vi "filters.vi"(4 "error in (no error)":errorcluster, 7 "Array":waveform(i16)[](array[waveform])) -> (3 "Array 2":waveform(i16)[](array[waveform]))   [LabVIEW 2010]
uses:
  <vilib>/Analysis/3filter.llb/Filter Passband Type.ctl
  skil/lib/Global 2.vi
  <vilib>/Analysis/3filter.llb/Equi-Ripple HighPass (DBL).vi
  <vilib>/Analysis/3filter.llb/Bessel Filter (DBL).vi
  <vilib>/Waveform/WDTOps.llb/WDT Get Waveform Subset I16.vi
  <vilib>/Utility/config.llb/NI_LVConfig.lvlib
  <vilib>/Analysis/NI_AALBase.lvlib
panel:
  out "Waveform Graph":waveform(i16)[](graph)
  out "error out":errorcluster
  in  "order":i32=3
  in  "high_freq":dbl=500000.0 format="%#_4p"
  in  "stop_freq":dbl=350000.0 format="%#_4p"
  in  "taps":i32=500
  in  "filter":enum16{"none", "Гребёнка", "FIR", "Bessel"}(ring)
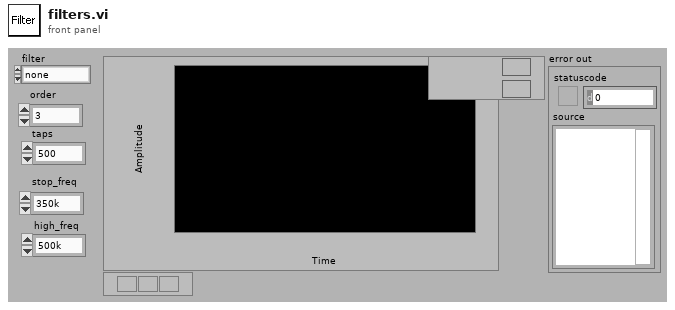
[diagram p1: front panel]
types:
  T1 = typedef "NI_AALBase.lvlib/Filter Passband Type.ctl" = enum32{"Lowpass", "Highpass", "Bandpass", "Bandstop"}
  T2 = typedef "NI_LVConfig.lvlib/Config Data RefNum.ctl" = refnum<k1>
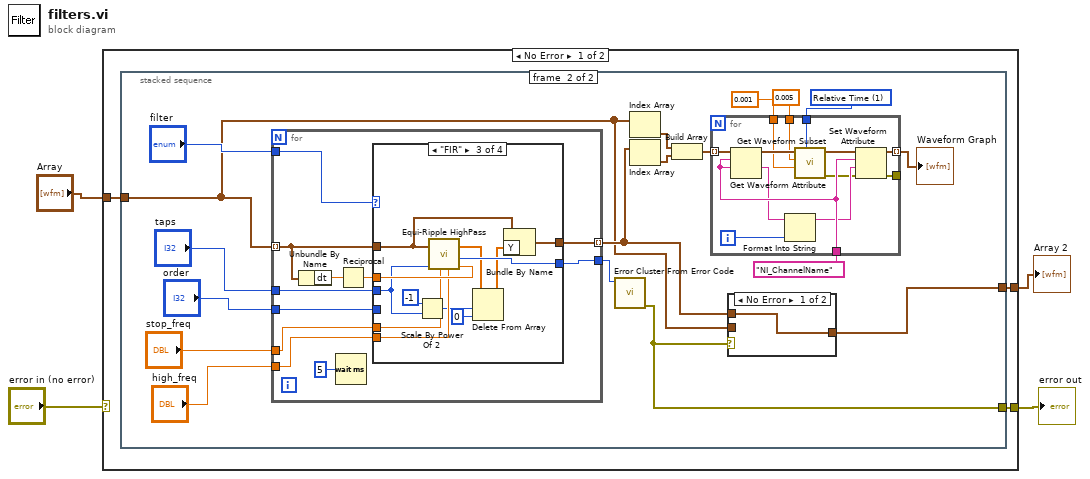
[diagram p0: block diagram]
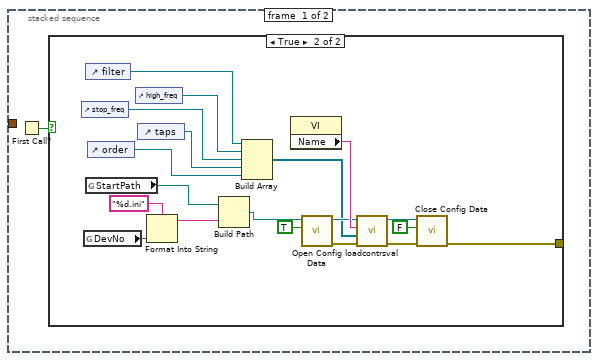
[diagram p2: hidden frame]
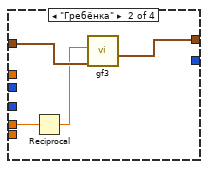
[diagram p6: hidden frame]
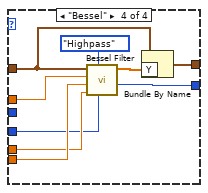
[diagram p7: hidden frame]
diagram:
  n1 = case shown="No Error" "error in (no error)" {
    selector: "error in (no error)" -> [_ w99]
    tunnel: [w7 w99] -> w3
    tunnel: "Array" -> [w6 w98]
    tunnel: [w5 w98] -> w1
    frame No Error {
      n2 = stacked-sequence {
        tunnel: [_ w31] -> w7
        tunnel: w6 -> [_ w29]
        tunnel: [_ w28] -> w5
        frame #0 {
          n3 = First Call?() -> (First Call?: T/F=w8:bool)
          n4 = case shown="True" w8 {
            tunnel: [_ w14] -> _
            frame False {
            }
            frame True {
              n5 = control-ref of="stop_freq"() -> (w11:refnum<vi>)
              n6 = global read "Global 2.vi" "DevNo"() -> (w18:i32)
              n7 = control-ref of="filter"() -> (w13:refnum<vi>)
              n8 = global read "Global 2.vi" "StartPath"() -> (w15:path)
              n9 = control-ref of="order"() -> (w9:refnum<vi>)
              n10 = control-ref of="high_freq"() -> (w12:refnum<vi>)
              n11 = control-ref of="taps"() -> (w10:refnum<vi>)
              n12 = Format Into String(format string="%d.ini", w18) -> (resulting string=w17:string)  [unwired: 2 in, 1 out]
              n13 = Build Path(base path=w15, name or relative path=w17) -> (appended path=w19:path)
              n14 = Build Array(w13, w12, w11, w10, w9) -> (w21:refnum<vi>[])
              n15 = property class="VI"() -> ("Name"=w24:string)  [unwired: 2 in, 2 out]
              n16 = call <vilib>:"Open Config Data.vi"("create file if necessary (T)"=TRUE, "configuration file path"=w19) -> ("error out"=w26:errorcluster, "refnum"=w23:T2)  [unwired: 7 in, 1 out]
              n17 = call "loadcontrsval.vi"("error in"=w26, "Array"=w21, "Section"=w24, "refnum in"=w23) -> ("error out"=w25:errorcluster, "refnum out"=w22:T2)  [unwired: 1 in, 1 out]
              n18 = call <vilib>:"Close Config Data.vi"("error in (no error)"=w25, "write file if changed (T)"=FALSE, "refnum"=w22) -> ("error out"=w14:errorcluster)  [unwired: 7 in, 1 out]
            }
          }
        }
        frame #1 {
          w39 = u16 1 items=["Index", "Relative Time"] ("start/duration format")
          n19 = for {
            tunnel: "filter" -> [w71]
            tunnel: w29 -> [w67] mode=indexing
            tunnel: [w70] -> w30 mode=indexing
            tunnel: [w69] -> w40
            tunnel: "taps" -> [w68]
            tunnel: "stop_freq" -> [w66]
            tunnel: "high_freq" -> [w65]
            tunnel: "order" -> [w64]
            n20 = Unbundle By Name(w67) -> ("dt"=w63:dbl)
            n21 = Wait (ms)(milliseconds to wait=u32 5) -> ()  [unwired: 1 out]
            n22 = Reciprocal(x=w63) -> (1/x=w62:dbl)
            n23 = case shown="\"FIR\"" w71 {
              tunnel: w67 -> [w72 w76 w84 w92]
              tunnel: [w72 w75 w83 w90] -> w70
              tunnel: [_ _ w88 w96] -> w69
              tunnel: w68 -> [_ _ w82 _]
              tunnel: w62 -> [_ _ w87 w95]
              tunnel: w66 -> [_ w74 w86 w93]
              tunnel: w65 -> [_ _ w85 w94]
              tunnel: w64 -> [_ _ _ w89]
              frame "none", Default {
              }
              frame "Гребёнка" {
                n24 = Reciprocal(x=w74) -> (1/x=w73:dbl)
                n25 = call "gf3.vi"("Waveform"=w76, "T"=w73) -> ("Waveform 2"=w75:waveform(i16))  [unwired: 4 in, 1 out]
              }
              frame "FIR" {
                n26 = Scale By Power Of 2(n=-1, x=w82) -> (x*2^n=w80:i32)
                n27 = call-poly <vilib>:"Equi-Ripple HighPass.vi"("# of taps"=w82, "stop freq"=w86, "high freq"=w85, "sampling freq: fs"=w87, "X"=w84) -> ("error"=w88:i32, "Filtered X"=w79:dbl[])  [unwired: 1 in]
                n28 = Delete From Array(array=w79, length=w80, index=0) -> (array with subset deleted=w78:dbl[])  [unwired: 1 out]
                n29 = Bundle By Name(cluster=w84, "Y"=w78) -> (w83:waveform(i16))
              }
              frame "Bessel" {
                n30 = call-poly <vilib>:"Bessel Filter.vi"("order"=w89, "filter type"=Filter_Passband_Type."Highpass", "low cutoff freq: fl"=w93, "high cutoff freq: fh"=w94, "sampling freq: fs"=w95, "X"=w92) -> ("error"=w96:i32, "Filtered X"=w91:dbl[])  [unwired: 2 in]
                n31 = Bundle By Name(cluster=w92, "Y"=w91) -> (w90:waveform(i16))
              }
            }
          }
          n32 = call <vilib>:"Error Cluster From Error Code.vi"("error code (0)"=w40) -> ("error out"=w31:errorcluster)  [unwired: 8 in]
          n33 = Index Array(array=w29) -> (element=w36:waveform(i16))  [unwired: 1 in]
          n34 = Index Array(array=w30) -> (element=w35:waveform(i16))  [unwired: 1 in]
          n35 = Build Array(w36, w35) -> (w34:waveform(i16)[])
          n36 = for {
            tunnel: w34 -> [w59] mode=indexing
            tunnel: [w56] -> w32 mode=indexing
            tunnel: w39 -> [w60]
            tunnel: "NI_ChannelName" -> [w53]
            tunnel: 0.001 ("duration") -> [w54]
            tunnel: 0.005 ("duration") -> [w50]
            tunnel: [w48] -> _
            i -> [w55]
            n37 = Get Waveform Attribute(5:w53, 6:w53, 7:w59) -> (1:w52:string, 3:w58:waveform(i16))  [unwired: 1 in, 2 out]
            n38 = Format Into String(initial string=w52, w55) -> (resulting string=w51:string)  [unwired: 2 in, 1 out]
            n39 = call-poly <vilib>:"Get Waveform Subset.vi"("start/duration format"=w60, "duration"=w54, "start samples/time"=w50, "waveform in"=w58) -> ("error out"=w49:errorcluster, "waveform out"=w57:waveform(i16))  [unwired: 2 in, 2 out]
            n40 = Set Waveform Attribute(4:w49, 5:w51, 6:w53, 7:w57) -> (0:w48:errorcluster, 3:w56:waveform(i16))  [unwired: 1 out]
          }
          "Waveform Graph" <- w32
          n41 = case shown="No Error" w31 {
            tunnel: w30 -> [w46 _]
            tunnel: w29 -> [_ w47]
            tunnel: [w46 w47] -> w28
            frame No Error {
            }
            frame Error {
            }
          }
        }
      }
    }
    frame Error {
    }
  }
  "error out" <- w3
  "Array 2" <- w1
